vi "AFM_Driver_Manager.Initialize.vi"(8 "error in (no error)":errorcluster, 11 "AFM_Driver_Manager in":refnum<class "AFM_Driver_Manager.lvclass">) -> (0 "error out":errorcluster, 3 "AFM_Driver_Manager out":refnum<class "AFM_Driver_Manager.lvclass">)   [LabVIEW 2019, in "AFM_Driver_Manager.lvclass"]
uses:
  AFM_Driver_Manager.lvclass
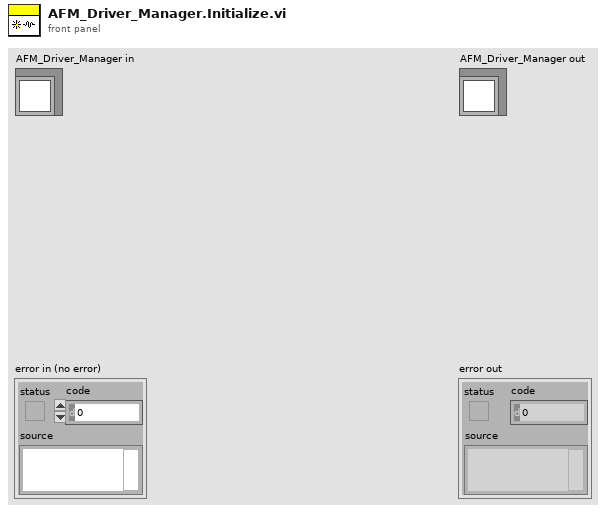
[diagram p1: front panel]
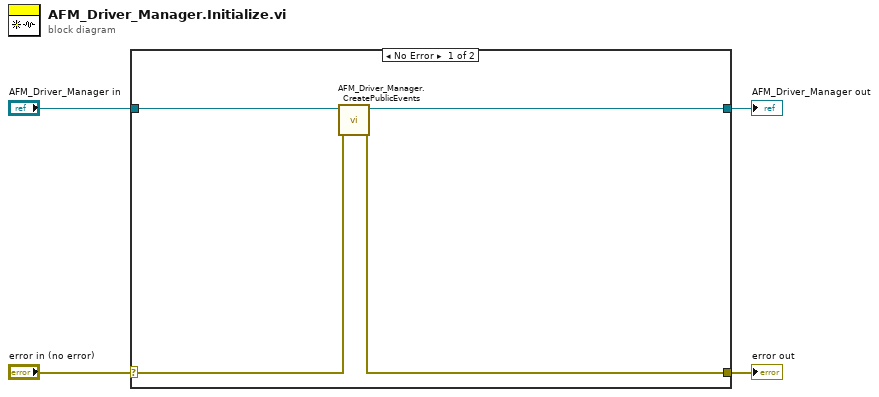
[diagram p0: block diagram]
diagram:
  n1 = case shown="No Error" "error in (no error)" {
    selector: "error in (no error)" -> [w6 w10]
    tunnel: [w5 w10] -> w3
    tunnel: [w8 w9] -> w1
    tunnel: "AFM_Driver_Manager in" -> [w7 w9]
    frame No Error {
      n2 = call "AFM_Driver_Manager.CreatePublicEvents.vi"("error in (no error)"=w6, "AFM_Driver_Manager in"=w7) -> ("error out"=w5:errorcluster, "AFM_Driver_Manager out"=w8:refnum<class "AFM_Driver_Manager.lvclass">)  [unwired: 8 in]
    }
    frame Error {
    }
  }
  "error out" <- w3
  "AFM_Driver_Manager out" <- w1
